vi "DP-Get F2 List.vi"(8 "error in (no error)":errorcluster, 11 "Comparison list":T1) -> (0 "error out":errorcluster, 3 "F2 List":string[](array[string]))   [LabVIEW 2020]
uses:
  Typedefs/DP-Comparison List.ctl
  <vilib>/Analysis/polynomials.llb/Unique Numbers and Multiplicity (DBL).vi
  <vilib>/Analysis/NI_AALPro.lvlib
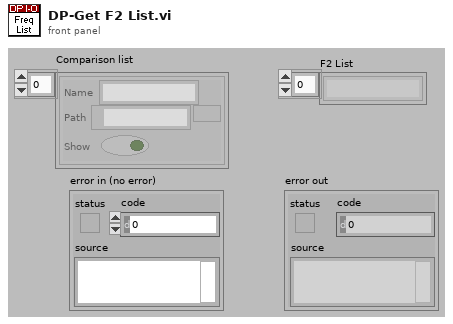
[diagram p1: front panel]
types:
  T1 = typedef "DP-Comparison List.ctl" = cluster{"Name":string, "Path":path, "Show":bool}[]
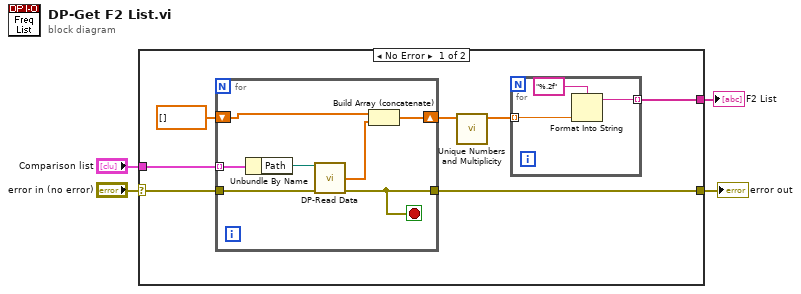
[diagram p0: block diagram]
diagram:
  n1 = case shown="No Error" "error in (no error)" {
    selector: "error in (no error)" -> [w7 w22]
    tunnel: "Comparison list" -> [w11 _]
    tunnel: [w8 w22] -> w3
    tunnel: [w5 _] -> w1
    frame No Error {
      n2 = for {
        tunnel: w11 -> [w21] mode=indexing
        tunnel: w7 -> [w19]
        shift-right: [w17] -> w9
        shift-left: dbl[] [] -> [w16]
        tunnel: [w15] -> w8
        stop <- w15 stop-if-true
        n3 = Unbundle By Name(w21) -> ("Path"=w20:path)
        n4 = call "DP-Read Data.vi"("Path"=w20, "error in"=w19) -> ("F2 array"=w18:dbl[], "error out"=w15:errorcluster)  [unwired: 10 in, 2 out]
        n5 = Build Array (concatenate)(w16, w18) -> (w17:dbl[])
      }
      n6 = call-poly <vilib>:"Unique Numbers and Multiplicity.vi"("Numbers"=w9) -> ("Unique Numbers"=w6:dbl[])  [unwired: 8 in, 2 out]
      n7 = for {
        tunnel: w6 -> [w14] mode=indexing
        tunnel: [w12] -> w5 mode=indexing
        n8 = Format Into String(format string="%.2f", w14) -> (resulting string=w12:string)  [unwired: 2 in, 1 out]
      }
    }
    frame Error {
    }
  }
  "error out" <- w3
  "F2 List" <- w1
